vi "plots.vi"   [LabVIEW 2012]
uses:
  <vilib>/addons/internet/NI_InternetTK_Core_VIs.lvlib
  <vilib>/addons/internet/NI_InternetTK_Common_VIs.lvlib
types:
  T1 = typedef "CGI Connection Info.ctl" = cluster{"name":string, "type":T2, "session":T3}
  T2 = typedef "CGI Request Type.ctl" = enum16{"cgi", ".spool first", ".spool", ".spool last"}
  T3 = typedef "HTTP Session.ctl" = refnum<k1>
  T4 = typedef "NI_FTP.lvlib/Keyed Array.ctl" = cluster{"keys":string[], "values":string[]}
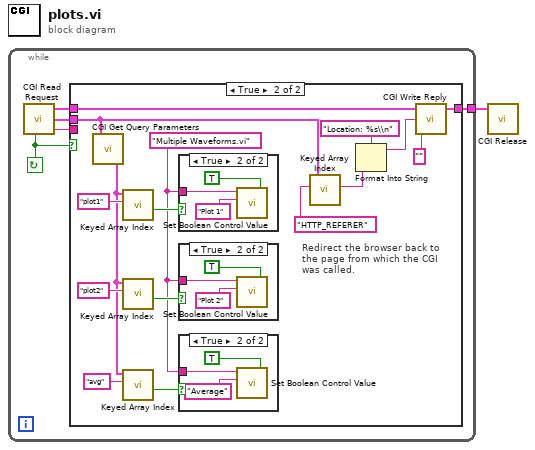
[diagram p0: block diagram]
diagram:
  n1 = while {
    tunnel: [w5] -> w1
    stop <- w4 continue-if-true
    n2 = call <vilib>:"CGI Read Request.vi"() -> ("valid request?"=w4:bool, "cgi connection info"=w6:T1, "env"=w3:T4, "content"=w2:string)  [unwired: 4 in]
    n3 = case shown="True" w4 {
      tunnel: [w7 w23] -> w5
      tunnel: w6 -> [w7 w22]
      tunnel: w3 -> [_ w13]
      tunnel: w2 -> [_ _]
      frame False {
      }
      frame True {
        w15 = "Multiple Waveforms.vi" ("VI name")
        # "Redirect the browser back to the page from which the CGI was called."
        n4 = call <vilib>:"CGI Get Query Parameters.vi"("env"=w13) -> ("query params"=w14:T4)  [unwired: 2 out]
        n5 = call <vilib>:"Keyed Array Index.vi"("key"="plot1", "array in"=w14) -> ("valid key"=w20:bool)  [unwired: 3 in, 2 out]
        n6 = call <vilib>:"Keyed Array Index.vi"("key"="plot2", "array in"=w14) -> ("valid key"=w19:bool)  [unwired: 3 in, 2 out]
        n7 = call <vilib>:"Keyed Array Index.vi"("key"="avg", "array in"=w14) -> ("valid key"=w16:bool)  [unwired: 3 in, 2 out]
        n8 = case shown="True" w20 {
          tunnel: w15 -> [_ w32]
          frame False {
          }
          frame True {
            n9 = call "Set Boolean Control Value.vi"("toggle (F)"=TRUE, "Control Name"="Plot 1" ("Button Name"), "VI name"=w32) -> ()  [unwired: 4 in, 1 out]
          }
        }
        n10 = case shown="True" w19 {
          tunnel: w15 -> [_ w29]
          frame False {
          }
          frame True {
            n11 = call "Set Boolean Control Value.vi"("toggle (F)"=TRUE, "Control Name"="Plot 2" ("Button Name"), "VI name"=w29) -> ()  [unwired: 4 in, 1 out]
          }
        }
        n12 = case shown="True" w16 {
          tunnel: w15 -> [_ w26]
          frame False {
          }
          frame True {
            n13 = call "Set Boolean Control Value.vi"("toggle (F)"=TRUE, "Control Name"="Average" ("Button Name"), "VI name"=w26) -> ()  [unwired: 4 in, 1 out]
          }
        }
        n14 = call <vilib>:"Keyed Array Index.vi"("key"="HTTP_REFERER", "array in"=w13) -> ("value"=w10:string)  [unwired: 3 in, 2 out]
        n15 = Format Into String(format string="Location: %s\\n", w10) -> (resulting string=w9:string)  [unwired: 2 in, 1 out]
        n16 = call <vilib>:"CGI Write Reply.vi"("content"="", "header"=w9, "cgi connection info"=w22) -> ("cgi connection info out"=w23:T1)  [unwired: 2 in]
      }
    }
  }
  n17 = call <vilib>:"CGI Release.vi"("cgi connection info"=w1) -> ()  [unwired: 5 in]
